vi "WPI_EncoderStop.vi"(8 "error in (no error)":errorcluster, 11 "EncoderDevRef":T1={"DevStatus"={"status"=FALSE, "code"=0, "source"=""}, "EncoderIndex"=enum."Invalid", "CounterIndex"=enum."Ctr 1", "DistancePerCount"=2.0, "Decoding Type"=enum."4x"}) -> (0 "error out":errorcluster, 3 "EncoderDevRef":T1={"DevStatus"={"status"=FALSE, "code"=0, "source"=""}, "EncoderIndex"=enum."Invalid", "CounterIndex"=enum."Ctr 1", "DistancePerCount"=2.0, "Decoding Type"=enum."4x"})   [LabVIEW 2017]
doc: "Stops decoding the signals the encoder you specify returns. Use the Reset VI if you want to reset the count of the encoder.\n\nThis software is licensed. Open the labview\\readme\\WPI Robotics Library Open Source License.txt file for more information."
uses:
  <vilib>/Rock Robotics/WPI/Encoder/WPI_EncoderDevRef.ctl
  <vilib>/Rock Robotics/SystemInterfaces/Encoder/FPGA_EncoderIdx.ctl
  <vilib>/Rock Robotics/SystemInterfaces/Counter/FPGA_CounterCtrSystemIndex.ctl
  <vilib>/Rock Robotics/WPI/Encoder/WPI_EncoderType.ctl
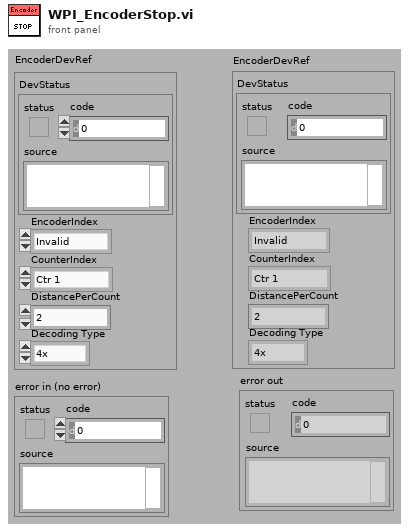
[diagram p1: front panel]
types:
  T1 = typedef "WPI_EncoderDevRef.ctl" = cluster{"DevStatus":errorcluster, "EncoderIndex":T2, "CounterIndex":T3, "DistancePerCount":dbl, "Decoding Type":T4}
  T2 = typedef "FPGA_EncoderIdx.ctl" = enum8{"Enc 0", "Enc 1", "Enc 2", "Enc 3", "Enc 4", "Enc 5", "Enc 6", "Enc 7", "Invalid"}
  T3 = typedef "FPGA_CounterCtrSystemIndex.ctl" = enum8{"Ctr 0", "Ctr 1", "Ctr 2", "Ctr 3", "Ctr 4", "Ctr 5", "Ctr 6", "Ctr 7", "Invalid"}
  T4 = typedef "WPI_EncoderType.ctl" = enum16{"1x", "2x", "4x"}
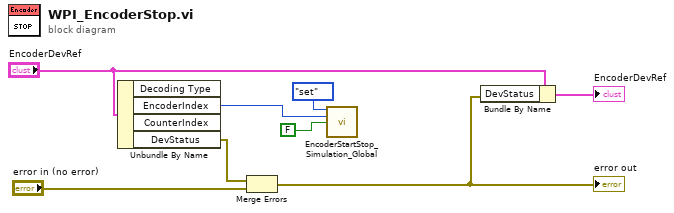
[diagram p0: block diagram]
diagram:
  n1 = Unbundle By Name("EncoderDevRef") -> ("EncoderIndex"=w1:T2, "DevStatus"=w5:errorcluster)  [unwired: 2 out]
  n2 = Merge Errors(w5, "error in (no error)") -> (w4:errorcluster)
  "error out" <- w4
  n3 = call <vilib>:"EncoderStartStop_Simulation_Global.vi"("menu"=enum16{"set", "get", "delete"}."set", "Encoder Index"=w1, "start/stop in"=FALSE ("Enable")) -> ()  [unwired: 11 in, 2 out]
  n4 = Bundle By Name(cluster="EncoderDevRef", "DevStatus"=w4) -> (→"EncoderDevRef":T1)
